vi "cv_07.vi"() -> ()   [LabVIEW 2013]
panel:
  in  "Knob":u8(knob) scale=0.0..10.0
  out "Numeric 3":dbl
  in  "Numeric 2":dbl
  in  "Numeric":dbl
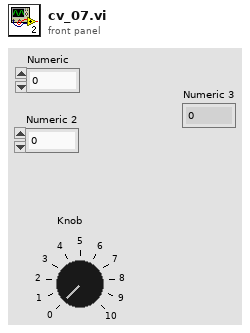
[diagram p1: front panel]
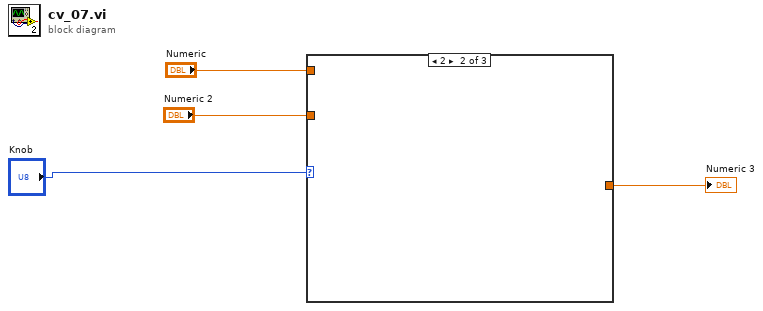
[diagram p0: block diagram]
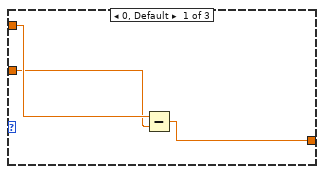
[diagram p2: hidden frame]
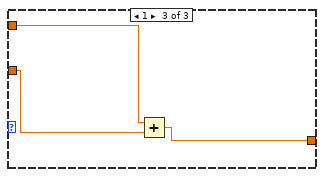
[diagram p3: hidden frame]
diagram:
  n1 = case shown="2" "Knob" {
    tunnel: "Numeric" -> [w7 _ w10]
    tunnel: "Numeric 2" -> [w6 _ w9]
    tunnel: [w5 _ w8] -> w2
    frame 0, Default {
      n2 = Subtract(x=w7, y=w6) -> (x-y=w5:dbl)
    }
    frame 2 {
    }
    frame 1 {
      n3 = Add(x=w10, y=w9) -> (x+y=w8:dbl)
    }
  }
  "Numeric 3" <- w2
